vi "WormQuantSingle.vi"() -> ()   [LabVIEW 2014]
uses:
  <vilib>/vision/NI_Vision_Development_Module.lvlib
panel:
  out "Video File:":string
  out "Motility Score":dbl=62758.35225749491
  out "Video Progress":u8(slide)=248
  out "Full Plate":T1(plugin-control)
  in  "Threshold":dbl=7.0
  in  "Step Size":i32=5 min=1
  # "By Timothy Kassis\nLast updated 11/15/14"
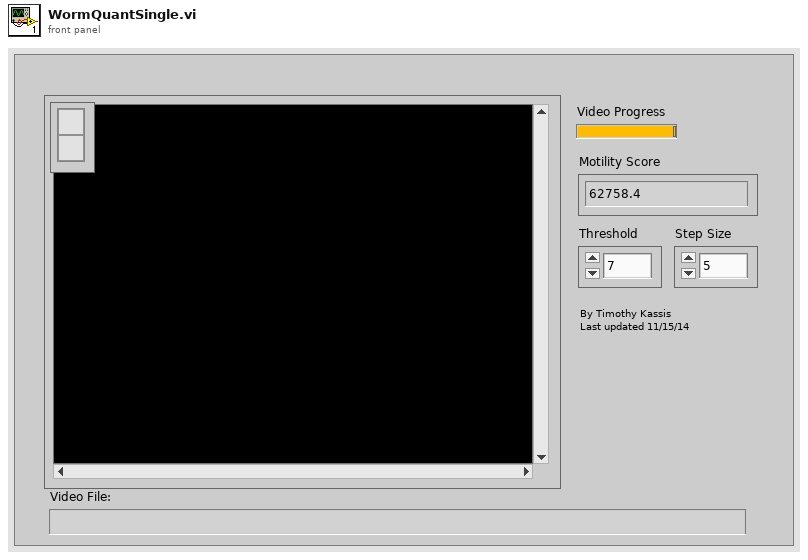
[diagram p1: front panel]
types:
  T1 = typedef "IMAQ Image.ctl" = refnum<image>
  T2 = typedef "Image Type" = u32
  T3 = typedef "IMAQ AVI2 Refnum.ctl" = refnum<k20>
  T4 = typedef "IMAQ Rectangle" = cluster{"Left":i32, "Top":i32, "Right":i32, "Bottom":i32, "Rotation":dbl}
  T5 = typedef "ROI Descriptor" = cluster{"Global Rectangle":i32[], "Contours":cluster{"ID":enum32{"External", "Internal"}, "Type":u32, "Coordinates":i32[]}[]}
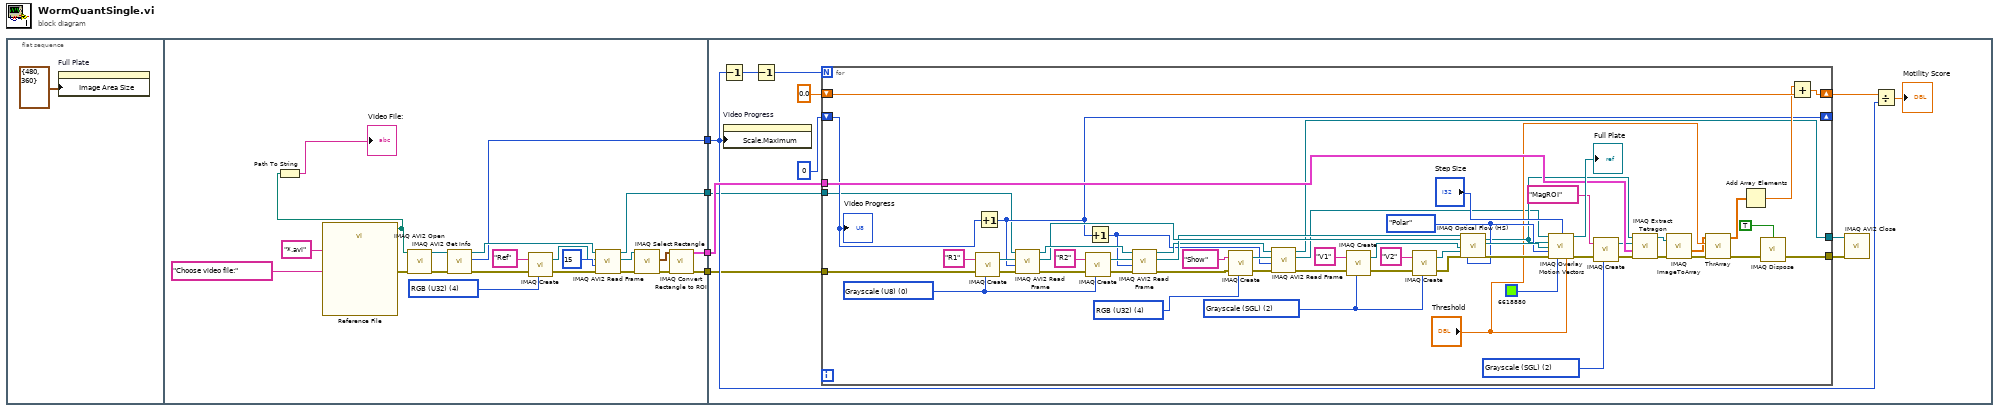
[diagram p0: block diagram]
diagram:
  n1 = flat-sequence {
    tunnel: [w14] -> w4
    tunnel: [w13] -> w3
    tunnel: [w10] -> w2
    tunnel: [w8] -> w1
    tunnel: w4 -> [w39]
    tunnel: w3 -> [w30]
    tunnel: w2 -> [w31]
    tunnel: w1 -> [w32]
    frame #0 {
      n2 = property on="Full Plate" class="ImageControl"("Image Area Size"=cluster{"Width":u32, "Height":u32} {"Width"=480, "Height"=360} ("Image Area:Size:All Elements")) -> ()  [unwired: 2 in, 2 out]
    }
    frame #1 {
      w25 = T2 4 items=["Grayscale (U8)", "Grayscale (I16)", "Grayscale (SGL)", "Complex (CSG)", "RGB (U32)", "HSL (U32)", "RGB (U64)", "Grayscale (U16)"] ("Image Type")
      n3 = call "Reference File"("prompt"="Choose video file:", "pattern (all files)"="*.avi") -> ("selected path"=w7:path, "error out"=w19:errorcluster)  [unwired: 10 in, 2 out]
      n4 = Path To String(path=w7) -> (string=→"Video File:":string)
      n5 = call "IMAQ AVI2 Open"("error in (no error)"=w19, "AVI File Path"=w7) -> ("error out"=w17:errorcluster, "AVI Refnum"=w18:T3)  [unwired: 8 in]
      n6 = call "IMAQ AVI2 Get Info"("error in (no error)"=w17, "AVI Refnum"=w18) -> ("error out"=w21:errorcluster, "Number of Frames"=w8:u32, "AVI Refnum (duplicate)"=w20:T3)  [unwired: 5 in, 2 out]
      n7 = call "IMAQ Create"("Image Name"="Ref", "Image Type"=w25, "error in (no error)"=w21) -> ("New Image"=w23:T1, "error out"=w22:errorcluster)  [unwired: 2 in]
      n8 = call "IMAQ AVI2 Read Frame"("error in (no error)"=w22, "Frame Number"=u32 15, "Image"=w23, "AVI Refnum"=w20) -> ("error out"=w9:errorcluster, "Image Out"=w26:T1, "AVI Refnum (duplicate)"=w10:T3)  [unwired: 5 in]
      n9 = call "IMAQ Select Rectangle"("error in (no error)"=w9, "Image In"=w26) -> ("error out"=w11:errorcluster, "Rectangle"=w12:T4)  [unwired: 6 in, 2 out]
      n10 = call "IMAQ Convert Rectangle to ROI"("error in (no error)"=w11, "Rectangle"=w12) -> ("error out"=w13:errorcluster, "ROI Descriptor"=w14:T5)  [unwired: 7 in]
    }
    frame #2 {
      n11 = Decrement(x=w32) -> (x-1=w34:u32)
      n12 = property on="Video Progress" class="Slide (strict)"("Scale.Maximum"=w32) -> ()  [unwired: 2 in, 2 out]
      n13 = Decrement(x=w34) -> (x-1=w35:u32)
      n14 = for {
        N: w35 -> [_]
        tunnel: [w87] -> w36
        tunnel: [w60] -> w37
        shift-right: [w66] -> _
        shift-left: 0 -> [w51]
        tunnel: w39 -> [w74]
        shift-right: [w68] -> w33
        shift-left: sgl 0.0 ("element") -> [w70]
        tunnel: w31 -> [w50]
        tunnel: w30 -> [w49]
        w40 = T2 2 items=["Grayscale (U8)", "Grayscale (I16)", "Grayscale (SGL)", "Complex (CSG)", "RGB (U32)", "HSL (U32)", "RGB (U64)", "Grayscale (U16)"] ("Image Type")
        w56 = T2 4 items=["Grayscale (U8)", "Grayscale (I16)", "Grayscale (SGL)", "Complex (CSG)", "RGB (U32)", "HSL (U32)", "RGB (U64)", "Grayscale (U16)"] ("Image Type")
        w73 = enum16{"Cartesian", "Polar"}."Polar" ("Velocity Representation")
        w64 = T2 2 items=["Grayscale (U8)", "Grayscale (I16)", "Grayscale (SGL)", "Complex (CSG)", "RGB (U32)", "HSL (U32)", "RGB (U64)", "Grayscale (U16)"] ("Image Type")
        w65 = T2 0 items=["Grayscale (U8)", "Grayscale (I16)", "Grayscale (SGL)", "Complex (CSG)", "RGB (U32)", "HSL (U32)", "RGB (U64)", "Grayscale (U16)"] ("Image Type")
        n15 = call "IMAQ Create"("Image Name"="R1", "Image Type"=w65, "error in (no error)"=w49) -> ("New Image"=w96:T1, "error out"=w79:errorcluster)  [unwired: 2 in]
        n16 = Increment(x=w51) -> (x+1=w66:i32)
        n17 = call "IMAQ AVI2 Read Frame"("error in (no error)"=w79, "Frame Number"=w66, "Image"=w96, "AVI Refnum"=w50) -> ("error out"=w78:errorcluster, "Image Out"=w82:T1, "AVI Refnum (duplicate)"=w92:T3)  [unwired: 5 in]
        n18 = call "IMAQ Create"("Image Name"="R2", "Image Type"=w65, "error in (no error)"=w78) -> ("New Image"=w93:T1, "error out"=w77:errorcluster)  [unwired: 2 in]
        n19 = Increment(x=w66) -> (x+1=w54:i32)
        n20 = call "IMAQ AVI2 Read Frame"("error in (no error)"=w77, "Frame Number"=w54, "Image"=w93, "AVI Refnum"=w92) -> ("error out"=w58:errorcluster, "Image Out"=w81:T1, "AVI Refnum (duplicate)"=w59:T3)  [unwired: 5 in]
        n21 = call "IMAQ Create"("Image Name"="Show", "Image Type"=w56, "error in (no error)"=w58) -> ("New Image"=w61:T1, "error out"=w62:errorcluster)  [unwired: 2 in]
        n22 = call "IMAQ AVI2 Read Frame"("error in (no error)"=w62, "Frame Number"=w54, "Image"=w61, "AVI Refnum"=w59) -> ("error out"=w57:errorcluster, "Image Out"=w55:T1, "AVI Refnum (duplicate)"=w60:T3)  [unwired: 5 in]
        n23 = call "IMAQ Create"("Image Name"="V1", "Image Type"=w64, "error in (no error)"=w57) -> ("New Image"=w83:T1, "error out"=w76:errorcluster)  [unwired: 2 in]
        n24 = call "IMAQ Create"("Image Name"="V2", "Image Type"=w64, "error in (no error)"=w76) -> ("New Image"=w84:T1, "error out"=w75:errorcluster)  [unwired: 2 in]
        n25 = call "IMAQ Optical Flow (HS)"("Current Frame"=w81, "Previous Frame"=w82, "Velocity Component 1 In"=w83, "Velocity Component 2 In"=w84, "error in (no error)"=w75, "Velocity Representation"=w73) -> ("Velocity Component 1 Out"=w72:T1, "Velocity Component 2 Out"=w80:T1, "error out"=w85:errorcluster)  [unwired: 10 in, 1 out]
        n26 = call "IMAQ Overlay Motion Vectors"("Image"=w55, "Step Size"="Step Size", "Velocity Component 1"=w72, "Velocity Component 2"=w80, "Velocity Representation"=w73, "error in (no error)"=w85, "Color"=u32 6618880, "Threshold"="Threshold") -> ("Image Out"=→"Full Plate":T1, "error out"=w71:errorcluster)  [unwired: 6 in]
        n27 = call "IMAQ Create"("Image Name"="MagROI", "Image Type"=w40, "error in (no error)"=w71) -> ("New Image"=w47:T1, "error out"=w48:errorcluster)  [unwired: 2 in]
        n28 = call-poly "IMAQ Extract Tetragon"("error in (no error)"=w48, "ROI Descriptor"=w74, "Image Dst"=w47, "Image Src"=w72) -> ("error out"=w45:errorcluster, "Image Dst Out"=w44:T1)  [unwired: 6 in]
        n29 = call "IMAQ ImageToArray"("error in (no error)"=w45, "Image"=w44) -> ("Image Pixels (Float)"=w43:sgl[][], "error out"=w41:errorcluster)  [unwired: 2 in, 3 out]
        n30 = call "ThrArray.vi"("Error In"=w41, "Threshold"="Threshold", "Input Array"=w43) -> ("Error Out"=w53:errorcluster, "Array"=w42:dbl[][])  [unwired: 7 in]
        n31 = Add Array Elements(numeric array=w42) -> (sum=w69:dbl)
        n32 = call "IMAQ Dispose"("All Images? (No)"=TRUE, "error in (no error)"=w53) -> ("error out"=w87:errorcluster)  [unwired: 4 in]
        n33 = Add(x=w69, y=w70) -> (x+y=w68:dbl)
        "Video Progress" <- w51
      }
      n34 = call "IMAQ AVI2 Close"("error in (no error)"=w36, "AVI Refnum"=w37) -> ()  [unwired: 9 in, 1 out]
      n35 = Divide(x=w33, y=w32) -> (x/y=→"Motility Score":dbl)
    }
  }
